vi "ke37xx System State.vi"(0 "VISA Resource Name":refnum<visa-resource-name>, 5 "Action":T1(ring), 9 "File Name":string, 11 "error in (no error)":errorcluster) -> (4 "VISA Resource Name Out":refnum<visa-resource-name>, 15 "error out":errorcluster)   [LabVIEW 2009, in "Keithley 3700 Series.lvlib"]
doc: "This VI allows you to save or recall saved system state information to/from internal memory or a file on a USB thumb drive."
uses:
  <instrlib>/Keithley 3706/Keithley 3700 Series.lvlib
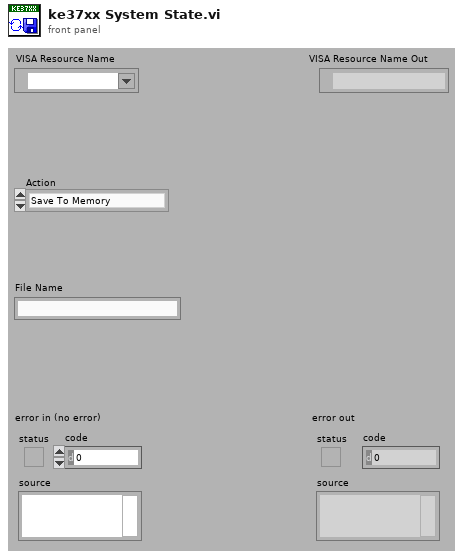
[diagram p1: front panel]
types:
  T1 = enum16{"Save To Memory", "Save To File", "Recall From Memory", "Recall From File"}
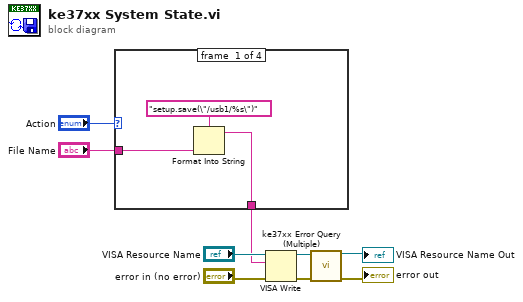
[diagram p0: block diagram]
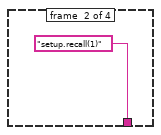
[diagram p2: hidden frame]
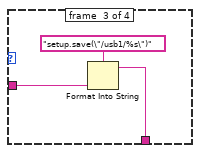
[diagram p3: hidden frame]
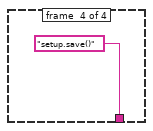
[diagram p4: hidden frame]
diagram:
  n1 = case shown="\"Recall From Memory\"" "Action" {
    tunnel: "File Name" -> [w11 _ w15 _]
    tunnel: [w10 "setup.recall(1)" w14 "setup.save()"] -> w1
    frame #0 {
      n2 = Format Into String(format string="setup.save(\"/usb1/%s\")", w11) -> (resulting string=w10:string)  [unwired: 2 in, 1 out]
    }
    frame #1 {
    }
    frame #2 {
      n3 = Format Into String(format string="setup.save(\"/usb1/%s\")", w15) -> (resulting string=w14:string)  [unwired: 2 in, 1 out]
    }
    frame #3 {
    }
  }
  n4 = VISA Write(VISA resource name="VISA Resource Name", write buffer=w1, error in (no error)="error in (no error)") -> (VISA resource name out=w5:refnum<visa-resource-name>, error out=w4:errorcluster)  [unwired: 1 out]
  n5 = call <instrlib>:"ke37xx Error Query (Multiple).vi"("VISA resource name"=w5, "error in (no error)"=w4) -> ("VISA resource name out"=→"VISA Resource Name Out":refnum<visa-resource-name>, "error out"=→"error out":errorcluster)  [unwired: 12 out]
